vi "hse-config-ini_OpenConfigSource.vi"(8 "error in (no error)":errorcluster, 11 "Name":string) -> (0 "error out":errorcluster, 2 "Config Data":T1, 3 "hse-config-ini out":refnum<class "hse-config-ini.lvclass">)   [LabVIEW 2022 SP3, in "hse-config-ini.lvclass"]
doc: "Finds the path to the <b>Name</b>.ini file inside the config/unit directory\n\n____\nHAMPEL SOFTWARE ENGINEERING v3.8.0 (2023-12-18 14:41)"
uses:
  hse-config-ini.lvclass
  hse-config-ini_ConfigData.ctl
  hse-application/hse-application.lvclass
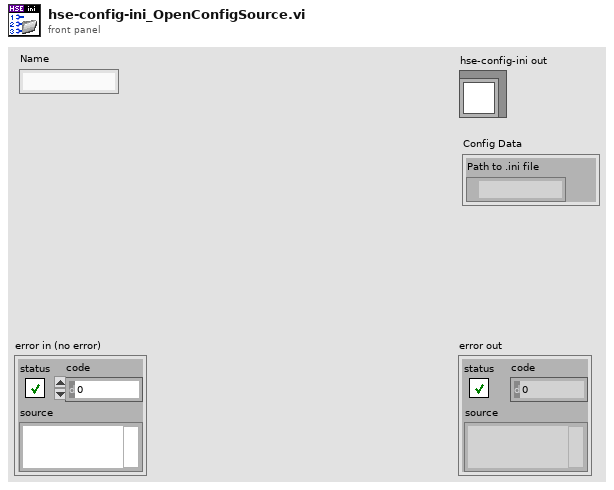
[diagram p1: front panel]
types:
  T1 = typedef "hse-config-ini.lvclass/hse-config-ini_ConfigData.ctl" = cluster{"Path to .ini file":path}
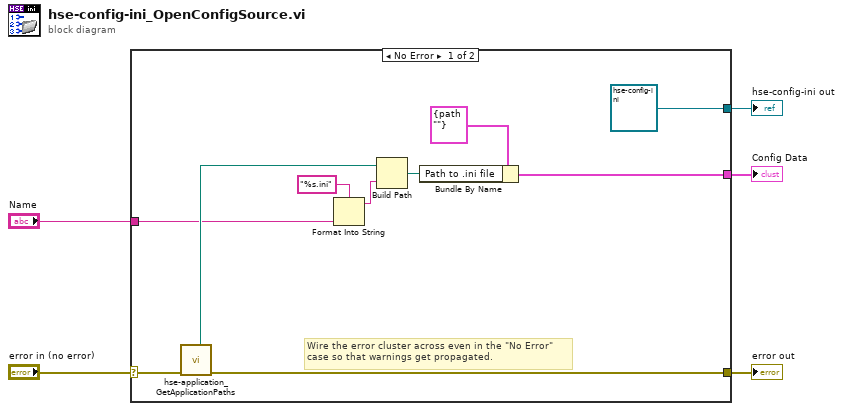
[diagram p0: block diagram]
diagram:
  n1 = case shown="No Error" "error in (no error)" {
    selector: "error in (no error)" -> [w8 w16]
    tunnel: [w7 w16] -> w4
    tunnel: [refnum<class "hse-config-ini.lvclass"> refnum ("hse-config-ini in") _] -> w3
    tunnel: "Name" -> [w6 _]
    tunnel: [w11 _] -> w1
    frame No Error {
      # "Wire the error cluster across even in the \"No Error\"\ncase so that warnings get propagated."
      n2 = call "hse-application_GetApplicationPaths.vi"("error in"=w8) -> ("error out"=w7:errorcluster, "Config/Unit Directory"=w9:path)  [unwired: 4 in, 5 out]
      n3 = Format Into String(format string="%s.ini", w6) -> (resulting string=w14:string)  [unwired: 2 in, 1 out]
      n4 = Build Path(base path=w9, name or relative path=w14) -> (appended path=w13:path)
      n5 = Bundle By Name(cluster=T1 {"Path to .ini file"=path ""} ("Config Data"), "Path to .ini file"=w13) -> (w11:T1)
    }
    frame Error {
    }
  }
  "error out" <- w4
  "hse-config-ini out" <- w3
  "Config Data" <- w1
